vi "VernierMove.vi"() -> ()   [LabVIEW 2019, in "Vernier.lvlib"]
uses:
  Vernier.lvlib
panel:
  out "Temperature":dbl
  out "Variation":dbl
  out "List 2":T1(ring)
  out "Custard6":dbl(slide) scale=0.0..50.0
  out "Custard5":dbl(slide) scale=0.0..50.0
  out "Custard4":dbl(slide) scale=0.0..50.0
  out "Custard3":dbl(slide) scale=0.0..50.0
  out "Custard2":dbl(slide) scale=0.0..50.0
  out "Custard1":dbl(slide) scale=0.0..50.0
  out "Waveform Chart":dbl[](graph)
  in  "List":T1(ring)
  in  "stop":bool
  out "OnHand":enum16{"Nothing", "PHSensor", "Temperature"}(ring)
  out "Doing":T1(ring)
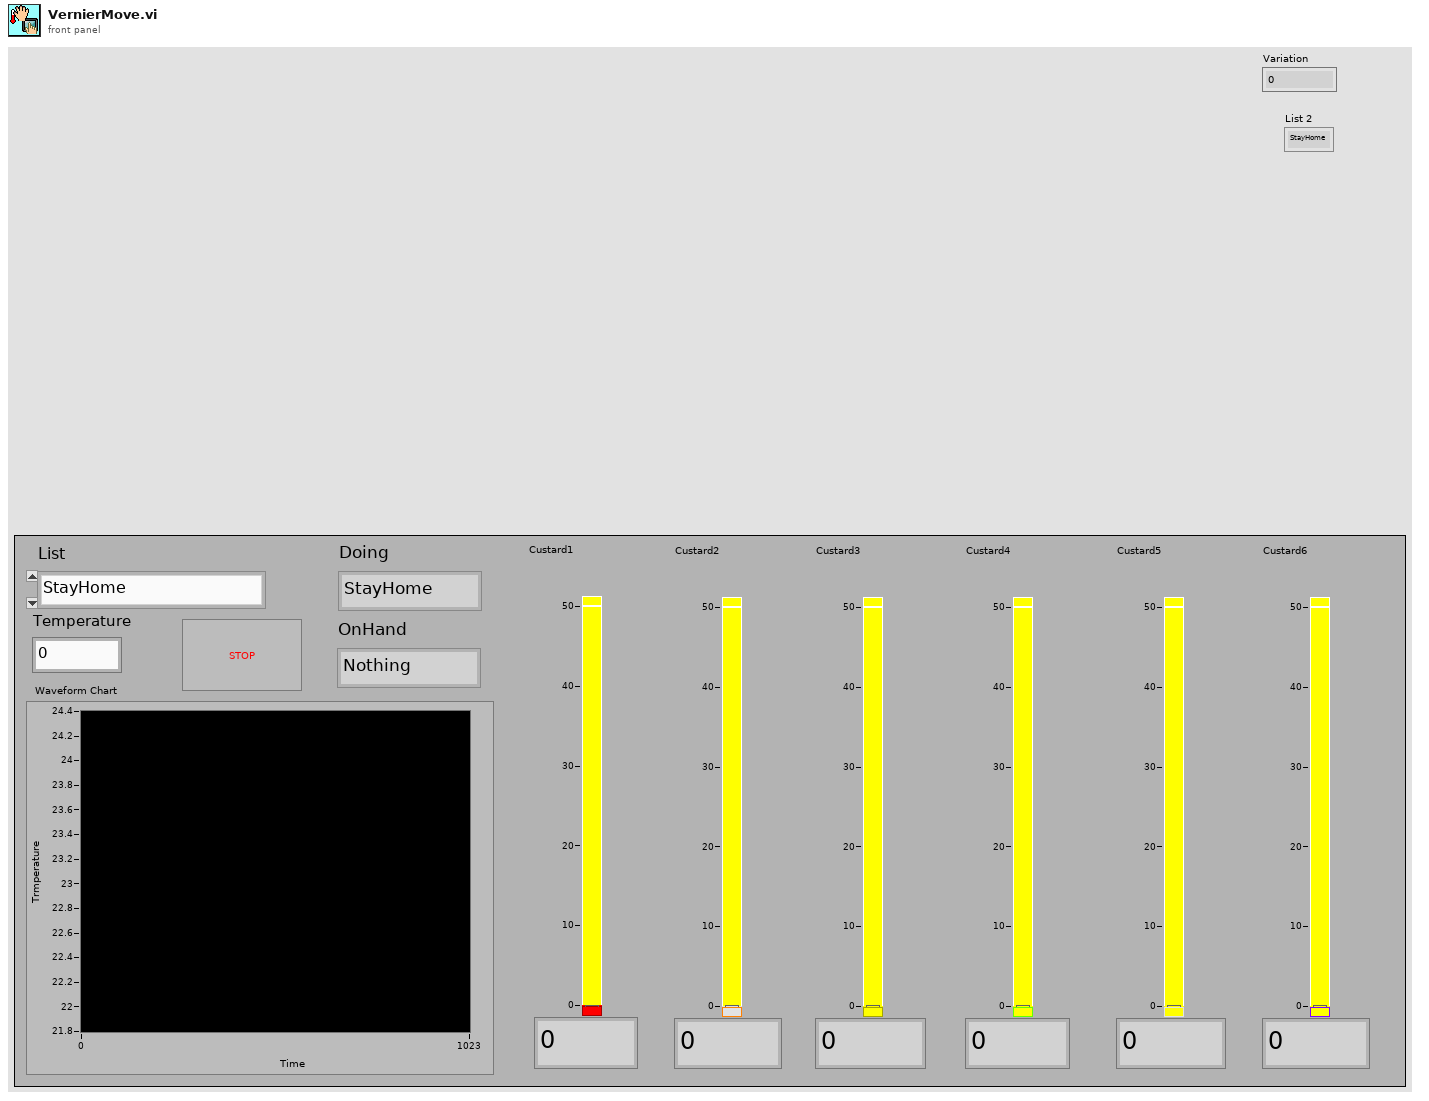
[diagram p1: front panel]
types:
  T1 = enum16{"StayHome", "Custard1", "Custard2", "Custard3", "Custard4", "Custard5", "Custard6", "PutBack", "SwtichPHSensor", "SwitchTemperature"}
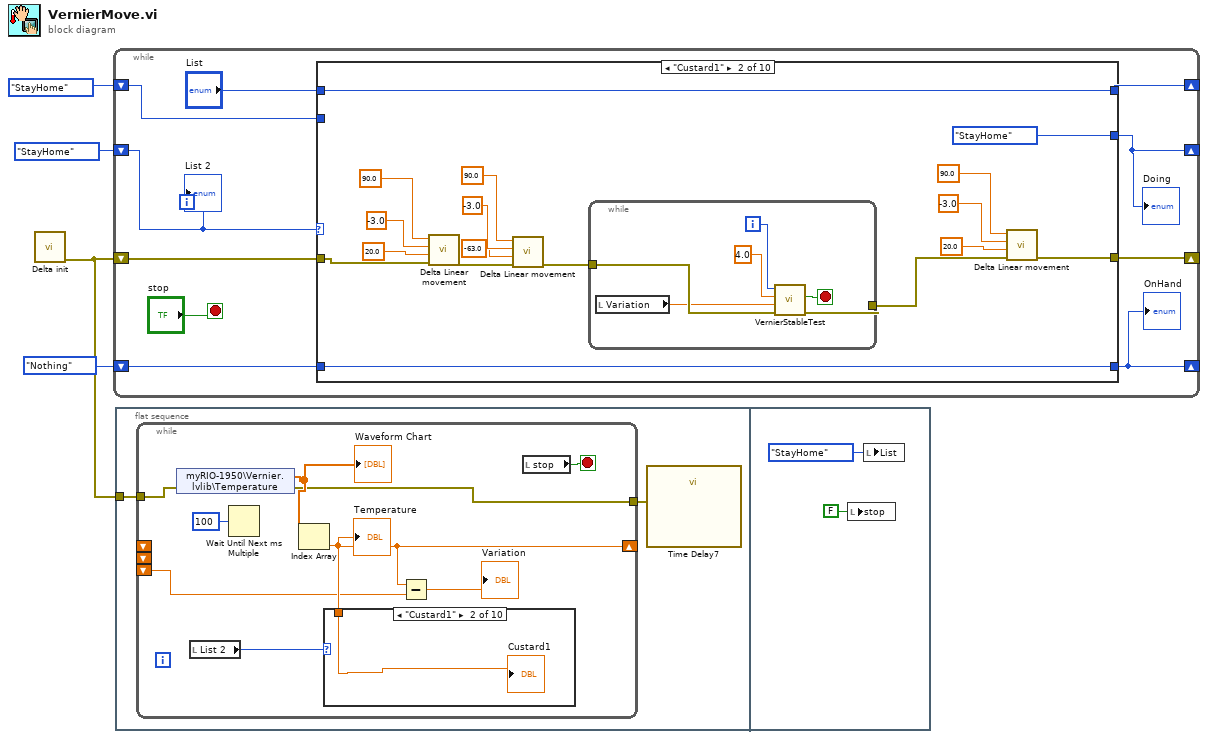
[diagram p0: block diagram]
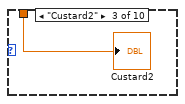
[diagram p3: hidden frame]
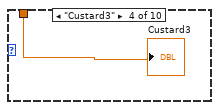
[diagram p4: hidden frame]
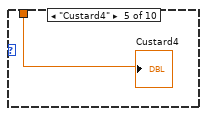
[diagram p5: hidden frame]
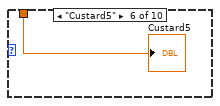
[diagram p6: hidden frame]
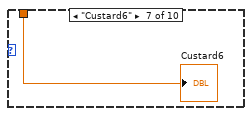
[diagram p7: hidden frame]
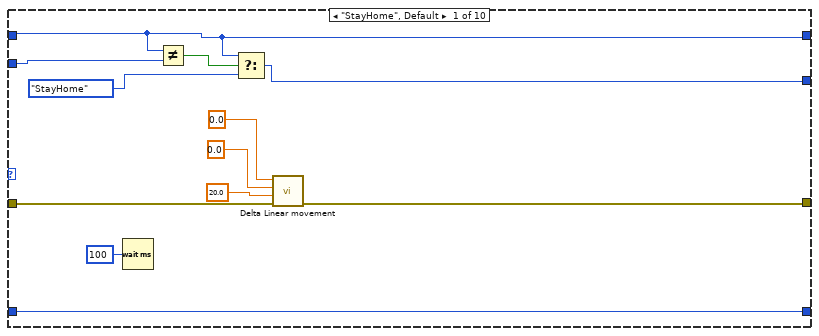
[diagram p11: hidden frame]
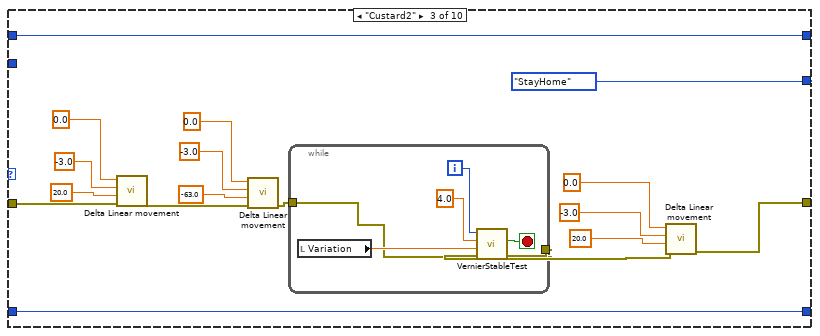
[diagram p12: hidden frame]
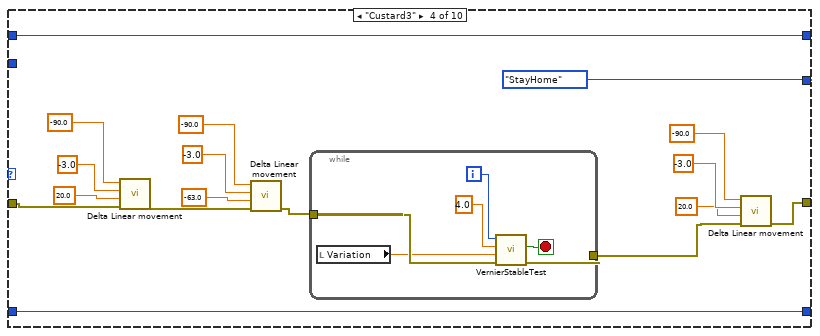
[diagram p13: hidden frame]
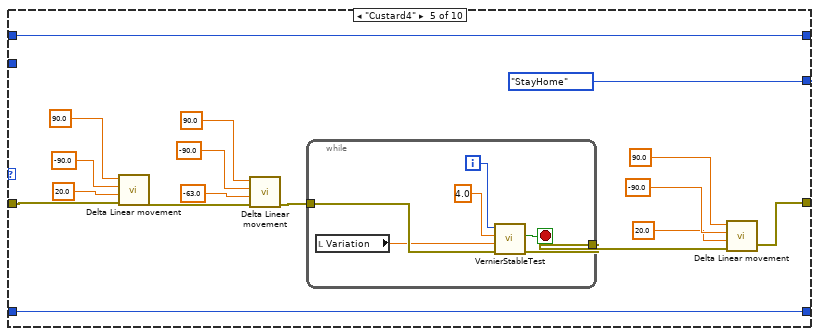
[diagram p14: hidden frame]
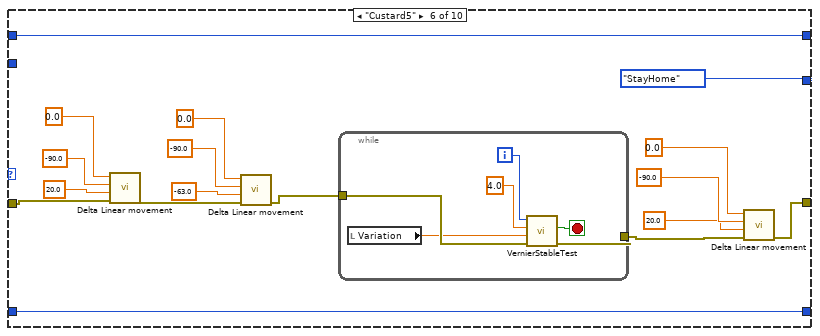
[diagram p15: hidden frame]
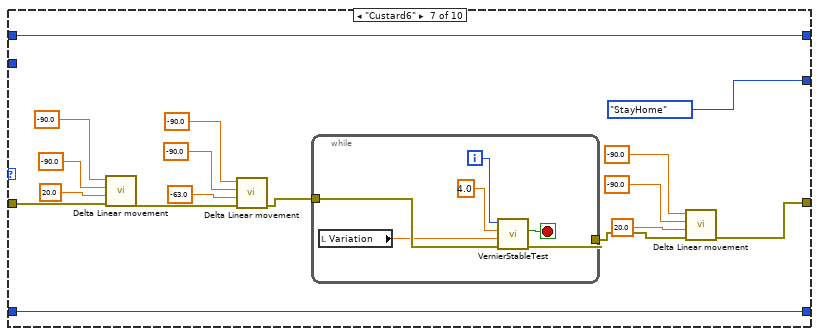
[diagram p16: hidden frame]
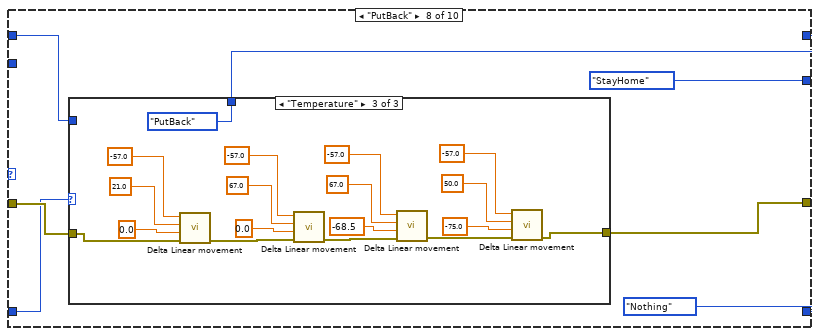
[diagram p17: hidden frame]
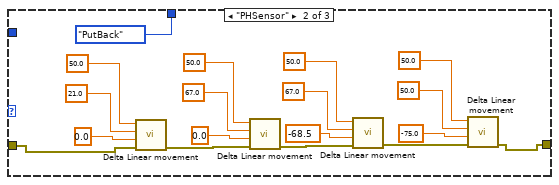
[diagram p19: hidden frame]
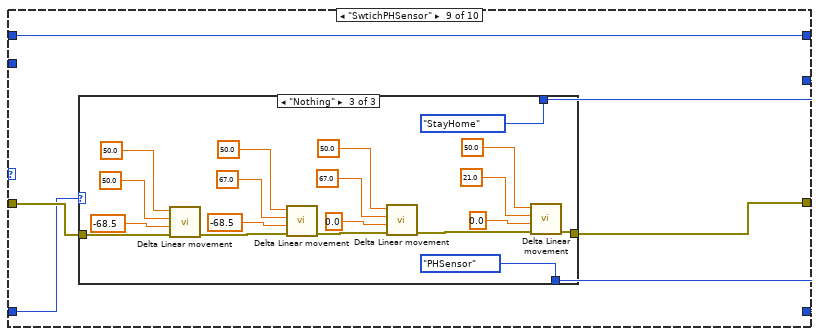
[diagram p20: hidden frame]
diagram:
  n1 = call "Delta init.vi"() -> ("error out"=w1:errorcluster)  [unwired: 9 in, 2 out]
  n2 = while {
    shift-right: [w6] -> _
    shift-left: T1."StayHome" ("List") -> [w14]
    shift-right: [w12] -> _
    shift-left: T1."StayHome" ("List") -> [w13]
    shift-right: [w11] -> _
    shift-left: w1 -> [w5]
    shift-right: [w10] -> _
    shift-left: enum16{"Nothing", "PHSensor", "Temperature"}."Nothing" ("Enum 2") -> [w9]
    stop <- "stop" stop-if-true
    n3 = case shown="\"Custard1\"" w14 {
      tunnel: "List" -> [w22 w43 w66 w89 w112 w135 w158 w165 w215 w244]
      tunnel: w5 -> [w26 w31 w53 w76 w99 w123 w146 w171 w214 w246]
      tunnel: [w22 w43 w66 w89 w112 w135 w158 w166 w215 w244] -> w12
      tunnel: w13 -> [w17 _ _ _ _ _ _ _ _ _]
      tunnel: [w20 w29 w52 w75 w98 w122 w145 w170 w210 w245] -> w11
      tunnel: [w21 w42 w65 w88 w111 w134 w157 enum16{"Nothing", "PHSensor", "Temperature"}."Nothing" ("Enum 2") w211 w241] -> w10
      tunnel: w9 -> [w21 w42 w65 w88 w111 w134 w157 w168 w213 w242]
      tunnel: [w16 T1."StayHome" ("Enum 2") T1."StayHome" ("Enum 2") T1."StayHome" ("Enum 2") T1."StayHome" ("Enum 2") T1."StayHome" ("Enum 2") T1."StayHome" ("Enum 2") T1."StayHome" ("Enum 2") w212 w243] -> w6
      frame "StayHome", Default {
        n4 = Wait (ms)(milliseconds to wait=u32 100) -> ()  [unwired: 1 out]
        n5 = Not Equal?(x=w22, y=w17) -> (x != y?=w18:bool)
        n6 = Select(t=w22, s=w18, f=T1."StayHome" ("Enum 2")) -> (s? t:f=w16:T1)
        n7 = call "Delta Linear movement.vi"("error in (no error)"=w26, "z0"=20.0, "y0"=0.0, "x0"=0.0) -> ("error out"=w20:errorcluster)  [unwired: 7 in]
      }
      frame "Custard1" {
        n8 = call "Delta Linear movement.vi"("error in (no error)"=w31, "z0"=20.0, "y0"=-3.0, "x0"=90.0) -> ("error out"=w35:errorcluster)  [unwired: 7 in]
        n9 = call "Delta Linear movement.vi"("error in (no error)"=w35, "z0"=-63.0, "y0"=-3.0, "x0"=90.0) -> ("error out"=w28:errorcluster)  [unwired: 7 in]
        n10 = while {
          tunnel: [w48] -> w27
          tunnel: w28 -> [w49]
          i -> [w44]
          stop <- w47 stop-if-true
          n11 = local read "Variation"() -> (w45:dbl)
          n12 = call "VernierStableTest.vi"("error in (no error)"=w49, "Custard"=w45, "Time Target (s)"=4.0, "i"=w44) -> ("error out"=w48:errorcluster, "Time has Elapsed"=w47:bool)  [unwired: 6 in]
        }
        n13 = call "Delta Linear movement.vi"("error in (no error)"=w27, "z0"=20.0, "y0"=-3.0, "x0"=90.0) -> ("error out"=w29:errorcluster)  [unwired: 7 in]
      }
      frame "Custard2" {
        n14 = call "Delta Linear movement.vi"("error in (no error)"=w53, "z0"=20.0, "y0"=-3.0, "x0"=0.0) -> ("error out"=w57:errorcluster)  [unwired: 7 in]
        n15 = call "Delta Linear movement.vi"("error in (no error)"=w57, "z0"=-63.0, "y0"=-3.0, "x0"=0.0) -> ("error out"=w51:errorcluster)  [unwired: 7 in]
        n16 = while {
          tunnel: [w72] -> w50
          tunnel: w51 -> [w67]
          i -> [w68]
          stop <- w71 stop-if-true
          n17 = local read "Variation"() -> (w69:dbl)
          n18 = call "VernierStableTest.vi"("error in (no error)"=w67, "Custard"=w69, "Time Target (s)"=4.0, "i"=w68) -> ("error out"=w72:errorcluster, "Time has Elapsed"=w71:bool)  [unwired: 6 in]
        }
        n19 = call "Delta Linear movement.vi"("error in (no error)"=w50, "z0"=20.0, "y0"=-3.0, "x0"=0.0) -> ("error out"=w52:errorcluster)  [unwired: 7 in]
      }
      frame "Custard3" {
        n20 = call "Delta Linear movement.vi"("error in (no error)"=w76, "z0"=20.0, "y0"=-3.0, "x0"=-90.0) -> ("error out"=w80:errorcluster)  [unwired: 7 in]
        n21 = call "Delta Linear movement.vi"("error in (no error)"=w80, "z0"=-63.0, "y0"=-3.0, "x0"=-90.0) -> ("error out"=w74:errorcluster)  [unwired: 7 in]
        n22 = while {
          tunnel: [w94] -> w73
          tunnel: w74 -> [w95]
          i -> [w90]
          stop <- w93 stop-if-true
          n23 = local read "Variation"() -> (w91:dbl)
          n24 = call "VernierStableTest.vi"("error in (no error)"=w95, "Custard"=w91, "Time Target (s)"=4.0, "i"=w90) -> ("error out"=w94:errorcluster, "Time has Elapsed"=w93:bool)  [unwired: 6 in]
        }
        n25 = call "Delta Linear movement.vi"("error in (no error)"=w73, "z0"=20.0, "y0"=-3.0, "x0"=-90.0) -> ("error out"=w75:errorcluster)  [unwired: 7 in]
      }
      frame "Custard4" {
        n26 = call "Delta Linear movement.vi"("error in (no error)"=w99, "z0"=20.0, "y0"=-90.0, "x0"=90.0) -> ("error out"=w103:errorcluster)  [unwired: 7 in]
        n27 = call "Delta Linear movement.vi"("error in (no error)"=w103, "z0"=-63.0, "y0"=-90.0, "x0"=90.0) -> ("error out"=w97:errorcluster)  [unwired: 7 in]
        n28 = while {
          tunnel: [w117] -> w96
          tunnel: w97 -> [w118]
          i -> [w113]
          stop <- w116 stop-if-true
          n29 = local read "Variation"() -> (w114:dbl)
          n30 = call "VernierStableTest.vi"("error in (no error)"=w118, "Custard"=w114, "Time Target (s)"=4.0, "i"=w113) -> ("error out"=w117:errorcluster, "Time has Elapsed"=w116:bool)  [unwired: 6 in]
        }
        n31 = call "Delta Linear movement.vi"("error in (no error)"=w96, "z0"=20.0, "y0"=-90.0, "x0"=90.0) -> ("error out"=w98:errorcluster)  [unwired: 7 in]
      }
      frame "Custard5" {
        n32 = call "Delta Linear movement.vi"("error in (no error)"=w123, "z0"=20.0, "y0"=-90.0, "x0"=0.0) -> ("error out"=w127:errorcluster)  [unwired: 7 in]
        n33 = call "Delta Linear movement.vi"("error in (no error)"=w127, "z0"=-63.0, "y0"=-90.0, "x0"=0.0) -> ("error out"=w120:errorcluster)  [unwired: 7 in]
        n34 = while {
          tunnel: [w140] -> w119
          tunnel: w120 -> [w141]
          i -> [w136]
          stop <- w139 stop-if-true
          n35 = local read "Variation"() -> (w137:dbl)
          n36 = call "VernierStableTest.vi"("error in (no error)"=w141, "Custard"=w137, "Time Target (s)"=4.0, "i"=w136) -> ("error out"=w140:errorcluster, "Time has Elapsed"=w139:bool)  [unwired: 6 in]
        }
        n37 = call "Delta Linear movement.vi"("error in (no error)"=w119, "z0"=20.0, "y0"=-90.0, "x0"=0.0) -> ("error out"=w122:errorcluster)  [unwired: 7 in]
      }
      frame "Custard6" {
        n38 = call "Delta Linear movement.vi"("error in (no error)"=w146, "z0"=20.0, "y0"=-90.0, "x0"=-90.0) -> ("error out"=w150:errorcluster)  [unwired: 7 in]
        n39 = call "Delta Linear movement.vi"("error in (no error)"=w150, "z0"=-63.0, "y0"=-90.0, "x0"=-90.0) -> ("error out"=w143:errorcluster)  [unwired: 7 in]
        n40 = while {
          tunnel: [w163] -> w142
          tunnel: w143 -> [w164]
          i -> [w159]
          stop <- w162 stop-if-true
          n41 = local read "Variation"() -> (w160:dbl)
          n42 = call "VernierStableTest.vi"("error in (no error)"=w164, "Custard"=w160, "Time Target (s)"=4.0, "i"=w159) -> ("error out"=w163:errorcluster, "Time has Elapsed"=w162:bool)  [unwired: 6 in]
        }
        n43 = call "Delta Linear movement.vi"("error in (no error)"=w142, "z0"=20.0, "y0"=-90.0, "x0"=-90.0) -> ("error out"=w145:errorcluster)  [unwired: 7 in]
      }
      frame "PutBack" {
        n44 = case shown="\"Temperature\"" w168 {
          tunnel: w171 -> [w173 w176 w194]
          tunnel: [w173 w175 w193] -> w170
          tunnel: [w172 T1."PutBack" ("Enum 2") T1."PutBack" ("Enum 2")] -> w166
          tunnel: w165 -> [w172 _ _]
          frame "Nothing", Default {
          }
          frame "PHSensor" {
            n45 = call "Delta Linear movement.vi"("error in (no error)"=w176, "z0"=0.0, "y0"=21.0, "x0"=50.0) -> ("error out"=w185:errorcluster)  [unwired: 7 in]
            n46 = call "Delta Linear movement.vi"("error in (no error)"=w185, "z0"=0.0, "y0"=67.0, "x0"=50.0) -> ("error out"=w178:errorcluster)  [unwired: 7 in]
            n47 = call "Delta Linear movement.vi"("error in (no error)"=w178, "z0"=-68.5, "y0"=67.0, "x0"=50.0) -> ("error out"=w177:errorcluster)  [unwired: 7 in]
            n48 = call "Delta Linear movement.vi"("error in (no error)"=w177, "z0"=-75.0, "y0"=50.0, "x0"=50.0) -> ("error out"=w175:errorcluster)  [unwired: 7 in]
          }
          frame "Temperature" {
            n49 = call "Delta Linear movement.vi"("error in (no error)"=w194, "z0"=0.0, "y0"=21.0, "x0"=-57.0) -> ("error out"=w203:errorcluster)  [unwired: 7 in]
            n50 = call "Delta Linear movement.vi"("error in (no error)"=w203, "z0"=0.0, "y0"=67.0, "x0"=-57.0) -> ("error out"=w196:errorcluster)  [unwired: 7 in]
            n51 = call "Delta Linear movement.vi"("error in (no error)"=w196, "z0"=-68.5, "y0"=67.0, "x0"=-57.0) -> ("error out"=w195:errorcluster)  [unwired: 7 in]
            n52 = call "Delta Linear movement.vi"("error in (no error)"=w195, "z0"=-75.0, "y0"=50.0, "x0"=-57.0) -> ("error out"=w193:errorcluster)  [unwired: 7 in]
          }
        }
      }
      frame "SwtichPHSensor" {
        n53 = case shown="\"Nothing\"" w213 {
          selector: w213 -> [w216 w219 _]
          tunnel: w214 -> [w218 w221 w223]
          tunnel: [w218 w221 w222] -> w210
          tunnel: [T1."StayHome" ("Enum 2") T1."PutBack" ("Enum 2") T1."StayHome" ("Enum 2")] -> w212
          tunnel: [w216 w219 enum16{"Nothing", "PHSensor", "Temperature"}."PHSensor" ("Enum 2")] -> w211
          frame "PHSensor" {
          }
          frame "Temperature" {
          }
          frame "Nothing" {
            n54 = call "Delta Linear movement.vi"("error in (no error)"=w223, "z0"=-68.5, "y0"=50.0, "x0"=50.0) -> ("error out"=w232:errorcluster)  [unwired: 7 in]
            n55 = call "Delta Linear movement.vi"("error in (no error)"=w232, "z0"=-68.5, "y0"=67.0, "x0"=50.0) -> ("error out"=w225:errorcluster)  [unwired: 7 in]
            n56 = call "Delta Linear movement.vi"("error in (no error)"=w225, "z0"=0.0, "y0"=67.0, "x0"=50.0) -> ("error out"=w224:errorcluster)  [unwired: 7 in]
            n57 = call "Delta Linear movement.vi"("error in (no error)"=w224, "z0"=0.0, "y0"=21.0, "x0"=50.0) -> ("error out"=w222:errorcluster)  [unwired: 7 in]
          }
        }
      }
      frame "SwitchTemperature" {
        n58 = case shown="\"Nothing\", Default" w242 {
          selector: w242 -> [_ w266 w269]
          tunnel: w246 -> [w249 w267 w271]
          tunnel: [w248 w267 w271] -> w245
          tunnel: [T1."StayHome" ("Enum 2") T1."PutBack" ("Enum 2") T1."StayHome" ("Enum 2")] -> w243
          tunnel: [enum16{"Nothing", "PHSensor", "Temperature"}."Temperature" ("Enum 2") w266 w269] -> w241
          frame "Nothing", Default {
            n59 = call "Delta Linear movement.vi"("error in (no error)"=w249, "z0"=-68.5, "y0"=50.0, "x0"=-57.0) -> ("error out"=w258:errorcluster)  [unwired: 7 in]
            n60 = call "Delta Linear movement.vi"("error in (no error)"=w258, "z0"=-68.5, "y0"=67.0, "x0"=-57.0) -> ("error out"=w251:errorcluster)  [unwired: 7 in]
            n61 = call "Delta Linear movement.vi"("error in (no error)"=w251, "z0"=0.0, "y0"=67.0, "x0"=-57.0) -> ("error out"=w250:errorcluster)  [unwired: 7 in]
            n62 = call "Delta Linear movement.vi"("error in (no error)"=w250, "z0"=0.0, "y0"=21.0, "x0"=-57.0) -> ("error out"=w248:errorcluster)  [unwired: 7 in]
          }
          frame "PHSensor" {
          }
          frame "Temperature" {
          }
        }
      }
    }
    "Doing" <- w6
    "OnHand" <- w10
    "List 2" <- w14
  }
  n63 = flat-sequence {
    tunnel: w1 -> [w273]
    frame #0 {
      n64 = while {
        tunnel: w273 -> [w281]
        tunnel: [w279] -> w272
        shift-right: [w276] -> _
        shift-left: _ -> [_]
        shift-left: _ -> [_]
        shift-left: _ -> [w274]
        stop <- w282 stop-if-true
        n65 = shared-variable "myRIO-1950\\Vernier.lvlib\\Temperature"(error in=w281) -> (w280:dbl[], error out=w279:errorcluster)
        "Waveform Chart" <- w280
        n66 = local read "List 2"() -> (w277:T1)
        n67 = Wait Until Next ms Multiple(millisecond multiple=u32 100) -> ()  [unwired: 1 out]
        n68 = Index Array(array=w280) -> (element=w276:dbl)  [unwired: 1 in]
        "Temperature" <- w276
        n69 = case shown="\"Custard1\"" w277 {
          tunnel: w276 -> [_ w283 w284 w285 w286 w287 w288 _ _ _]
          frame "StayHome", Default {
          }
          frame "Custard1" {
            "Custard1" <- w283
          }
          frame "Custard2" {
            "Custard2" <- w284
          }
          frame "Custard3" {
            "Custard3" <- w285
          }
          frame "Custard4" {
            "Custard4" <- w286
          }
          frame "Custard5" {
            "Custard5" <- w287
          }
          frame "Custard6" {
            "Custard6" <- w288
          }
          frame "PutBack" {
          }
          frame "SwtichPHSensor" {
          }
          frame "SwitchTemperature" {
          }
        }
        n70 = Subtract(x=w276, y=w274) -> (x-y=→"Variation":dbl)
        n71 = local read "stop"() -> (w282:bool)
      }
      n72 = call "Time Delay7"("error in (no error)"=w272) -> ()  [unwired: 10 in, 1 out]
    }
    frame #1 {
      n73 = local write "stop"(FALSE ("stop")) -> ()
      n74 = local write "List"(T1."StayHome" ("List")) -> ()
    }
  }
